vi "sub_DO-ch.vi"(7 "onoff":bool=TRUE, 8 "error in":errorcluster, 10 "pos":enum16{"input", "output"}(ring), 11 "현재채널번호":u8) -> (0 "error out":errorcluster)   [LabVIEW 2019]
uses:
  _ctrl/rw.ctl
  cnt_Relay.ctl
  _ctrl/start.ctl
  _ctrl/create-rw-close.ctl
  <vilib>/DAQmx/write.llb/DAQmx Write (Digital Bool 1Line 1Point).vi
  Durability/common/Global 1.vi
  <vilib>/DAQmx/create/channels.llb/DAQmx Create Channel (DO-Digital Output).vi
  <vilib>/DAQmx/miscellaneous.llb/DAQmx Fill In Error Info.vi
panel:
  out "ch name full":string
  out "in-out":bool
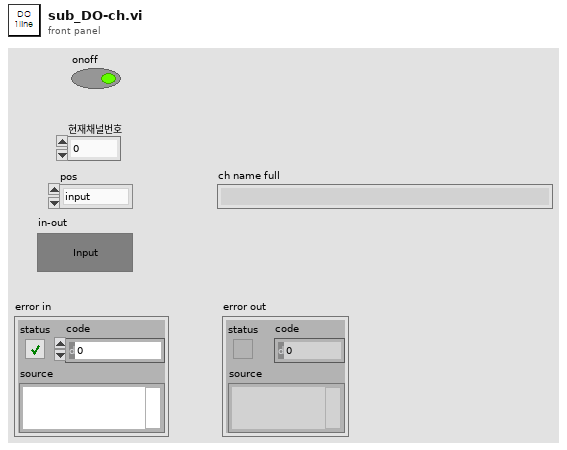
[diagram p1: front panel]
types:
  T1 = typedef "rw.ctl" = enum16{"read", "write"}
  T2 = typedef "start.ctl" = enum16{"init", "open", "set", "start", "stop", "read", "read_items", "query", "close", "T_single", "reset", "exit"}
  T3 = typedef "create-rw-close.ctl" = enum16{"create", "write", "read", "delete", "close"}
  T4 = typedef "cnt_Relay.ctl" = enum32{"R_Load", "R_out1", "R_out2", "R_out3", "R_out4", "R_out5", "R_out6", "R8", "R9", "R10", "R11", "R12", "R13", "R14", "R15", "R16", "R_in1", "R_in2", "R_in3", "R_in4", "R_in5", "R_in6", "R23", "R24", "R25", "R26", "R27", "R_red", "R_yellow", "R_green", "R_buz", "R_purple"}
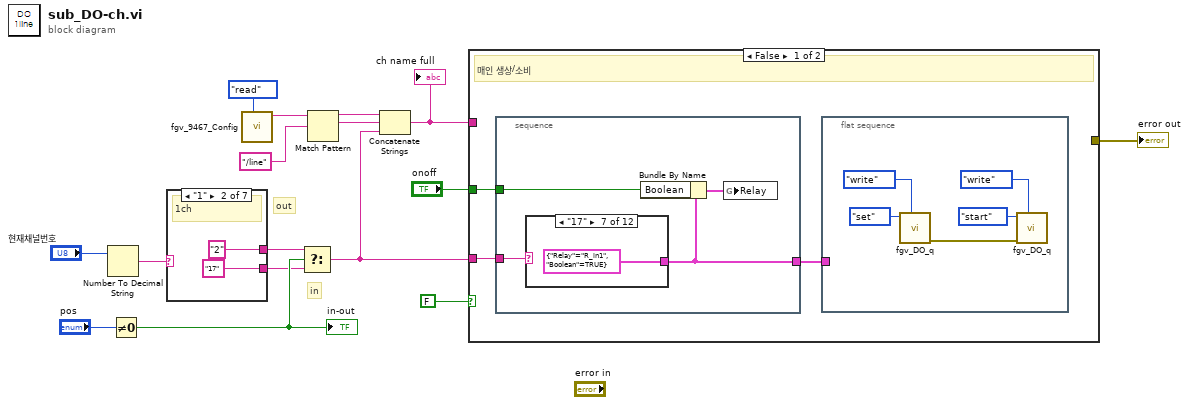
[diagram p0: block diagram]
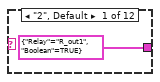
[diagram p2: hidden frame]
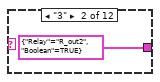
[diagram p3: hidden frame]
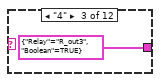
[diagram p4: hidden frame]
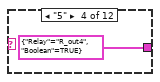
[diagram p5: hidden frame]
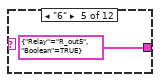
[diagram p6: hidden frame]
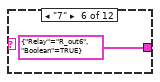
[diagram p7: hidden frame]
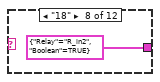
[diagram p8: hidden frame]
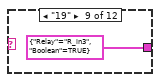
[diagram p9: hidden frame]
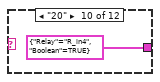
[diagram p10: hidden frame]
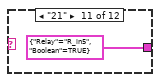
[diagram p11: hidden frame]
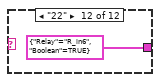
[diagram p12: hidden frame]
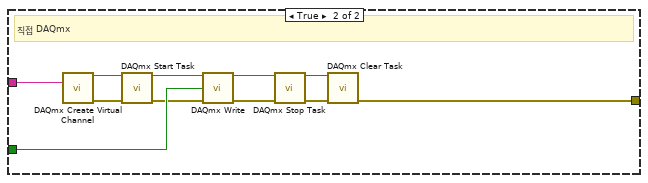
[diagram p13: hidden frame]
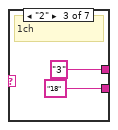
[diagram p15: hidden frame]
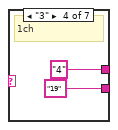
[diagram p16: hidden frame]
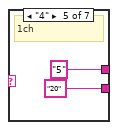
[diagram p17: hidden frame]
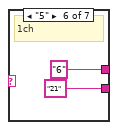
[diagram p18: hidden frame]
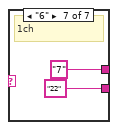
[diagram p19: hidden frame]
diagram:
  # "in"
  # "out"
  n1 = Number To Decimal String(number="현재채널번호") -> (decimal integer string=w13:string)  [unwired: 1 in]
  n2 = Not Equal To 0?(x="pos") -> (x != 0?=w5:bool)
  "in-out" <- w5
  n3 = case shown="\"1\"" w13 {
    tunnel: [_ "17" ("string") "18" ("string") "19" ("string") "20" ("string") "21" ("string") "22" ("string")] -> w3
    tunnel: [_ "2" ("string") "3" ("string") "4" ("string") "5" ("string") "6" ("string") "7" ("string")] -> w2
    frame "False", Default {
    }
    frame "1" {
      # "1ch"
    }
    frame "2" {
      # "1ch"
    }
    frame "3" {
      # "1ch"
    }
    frame "4" {
      # "1ch"
    }
    frame "5" {
      # "1ch"
    }
    frame "6" {
      # "1ch"
    }
  }
  n4 = call "fgv_9467_Config.vi"("cmd"=rw."read") -> ("cDAQ-9467 Config 2"=w10:tag)  [unwired: 10 in]
  n5 = Select(t=w2, s=w5, f=w3) -> (s? t:f=w1:string)
  n6 = Match Pattern(string=w10, regular expression="/line" ("string")) -> (before substring=w8:string, match substring=w7:string)  [unwired: 1 in, 2 out]
  n7 = Concatenate Strings(w8, w7, w1) -> (w12:string)
  "ch name full" <- w12
  n8 = case shown="False" FALSE {
    tunnel: "onoff" -> [w30 w63]
    tunnel: w12 -> [_ w54]
    tunnel: [_ w53] -> w11
    tunnel: w1 -> [w31 _]
    frame False {
      # "매인 생상/소비"
      n9 = stacked-sequence {
        tunnel: w31 -> [w40]
        tunnel: w30 -> [w39]
        tunnel: [w37] -> w29
        frame #0 {
          n10 = case shown="\"17\"" w40 {
            tunnel: [cluster{"Relay":T4, "Boolean":bool} {"Relay"=enum."R_out1", "Boolean"=TRUE} ("Relay") cluster{"Relay":T4, "Boolean":bool} {"Relay"=enum."R_out2", "Boolean"=TRUE} ("Relay") cluster{"Relay":T4, "Boolean":bool} {"Relay"=enum."R_out3", "Boolean"=TRUE} ("Relay") cluster{"Relay":T4, "Boolean":bool} {"Relay"=enum."R_out4", "Boolean"=TRUE} ("Relay") cluster{"Relay":T4, "Boolean":bool} {"Relay"=enum."R_out5", "Boolean"=TRUE} ("Relay") cluster{"Relay":T4, "Boolean":bool} {"Relay"=enum."R_out6", "Boolean"=TRUE} ("Relay") cluster{"Relay":T4, "Boolean":bool} {"Relay"=enum."R_in1", "Boolean"=TRUE} ("Relay") cluster{"Relay":T4, "Boolean":bool} {"Relay"=enum."R_in2", "Boolean"=TRUE} ("Relay") cluster{"Relay":T4, "Boolean":bool} {"Relay"=enum."R_in3", "Boolean"=TRUE} ("Relay") cluster{"Relay":T4, "Boolean":bool} {"Relay"=enum."R_in4", "Boolean"=TRUE} ("Relay") cluster{"Relay":T4, "Boolean":bool} {"Relay"=enum."R_in5", "Boolean"=TRUE} ("Relay") cluster{"Relay":T4, "Boolean":bool} {"Relay"=enum."R_in6", "Boolean"=TRUE} ("Relay")] -> w37
            frame "2", Default {
            }
            frame "3" {
            }
            frame "4" {
            }
            frame "5" {
            }
            frame "6" {
            }
            frame "7" {
            }
            frame "17" {
            }
            frame "18" {
            }
            frame "19" {
            }
            frame "20" {
            }
            frame "21" {
            }
            frame "22" {
            }
          }
          n11 = Bundle By Name(cluster=w37, "Boolean"=w39) -> (w38:cluster{"Relay":T4, "Boolean":bool})
          n12 = global write "Global 1.vi" "Relay"(w38) -> ()
        }
      }
      n13 = flat-sequence {
        tunnel: w29 -> [_]
        frame #0 {
          n14 = call "fgv_DO_q.vi"("cmd"=create-rw-close."write", "data"=start."set") -> ("error out"=w36:errorcluster)  [unwired: 8 in, 1 out]
          n15 = call "fgv_DO_q.vi"("cmd"=create-rw-close."write", "error in"=w36, "data"=start."start") -> ()  [unwired: 7 in, 2 out]
        }
      }
    }
    frame True {
      # "직접 DAQmx"
      n16 = call-poly <vilib>:"DAQmx Create Virtual Channel.vi"("lines"=w54) -> ("task out"=w61:refnum<k21>, "error out"=w62:errorcluster)  [unwired: 13 in]
      n17 = call <vilib>:"DAQmx Start Task.vi"("task/channels in"=w61, "error in"=w62) -> ("task out"=w58:refnum<k21>, "error out"=w57:errorcluster)  [unwired: 12 in]
      n18 = call-poly <vilib>:"DAQmx Write.vi"("task/channels in"=w58, "data"=w63, "error in"=w57) -> ("task out"=w56:refnum<k21>, "error out"=w55:errorcluster)  [unwired: 10 in, 1 out]
      n19 = call <vilib>:"DAQmx Stop Task.vi"("task/channels in"=w56, "error in"=w55) -> ("task out"=w60:refnum<k21>, "error out"=w59:errorcluster)  [unwired: 12 in]
      n20 = call <vilib>:"DAQmx Clear Task.vi"("task in"=w60, "error in"=w59) -> ("error out"=w53:errorcluster)  [unwired: 13 in]
    }
  }
  "error out" <- w11
